vi "Diagnostic.vi"(8 "error in (no error)":errorcluster, 11 "Connection Data In":T1) -> (0 "error out":errorcluster, 3 "Connection Data Out":T1)   [LabVIEW 2014, in "MSX-E3711_dll.lvlib"]
doc: "Encargado de Testear si hay transductores desconectados, si se produjo un corto circuito en alguno de ellos y de rearmarlos."
uses:
  MSX-E3711_dll.lvlib
  Typedef/Connection Data.ctl
  E:/Repositorio Magnis/INF002/v0/Modules/HAL/Drivers/Sync/ADDI-DATA MSX-E3711/API/MSXE371x.dll
  MSXE371x.dll
  E:/Repositorio Magnis/INF002/v0/Modules/HAL/Drivers/Sync/ADDI-DATA MSX-E3711/API/MXCommon.dll
  MXCommon.dll
panel:
  out "String":string
  out "Rearm \nTransducers Status":bool
  out "Progress Status":i32(slide) scale=0.0..100.0
  out "Table":string[][](table)=[["-", "-"], ["-", "-"], ["-", "-"], ["-", "-"], ["-", "-"], ["-", "-"], ["-", "-"], ["-", "-"], ["-", "-"], ["-", "-"], ["-", "-"], ["-", "-"], ["-", "-"], ["-", "-"], ["-", "-"], ["-", "-"], ["-", "-"]]
  in  "Rearm Transducers":bool
  in  "ConnectionStatus":bool
  in  "ShortCircuit":bool
  in  "Start":bool
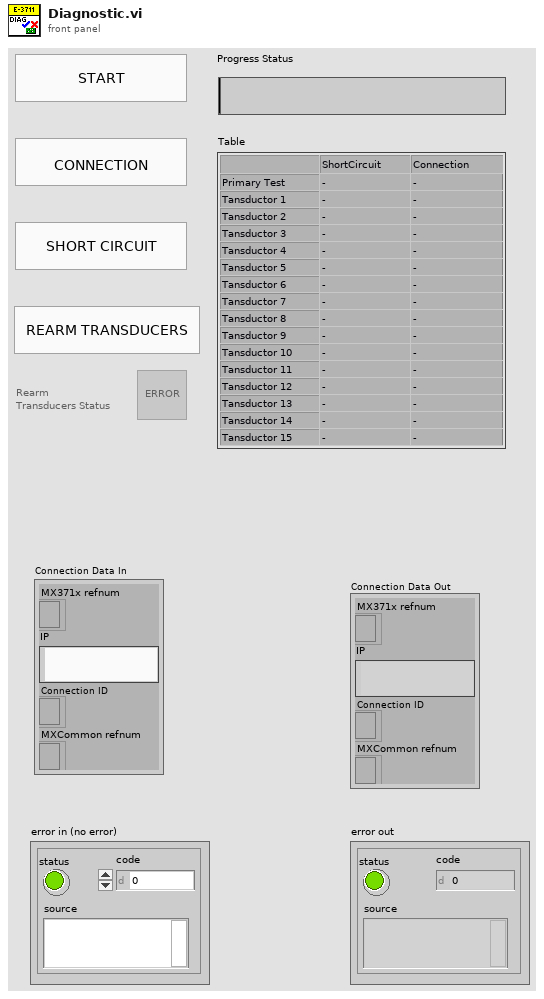
[diagram p1: front panel]
types:
  T1 = typedef "MSX-E3711_dll.lvlib/Connection Data.ctl" = cluster{"MX371x refnum":refnum<k24>, "IP":string, "Connection ID ":refnum<k5>, "MXCommon refnum":refnum<k24>}
  T2 = enum8{"Enabled", "Disabled", "Disabled and Grayed Out"}
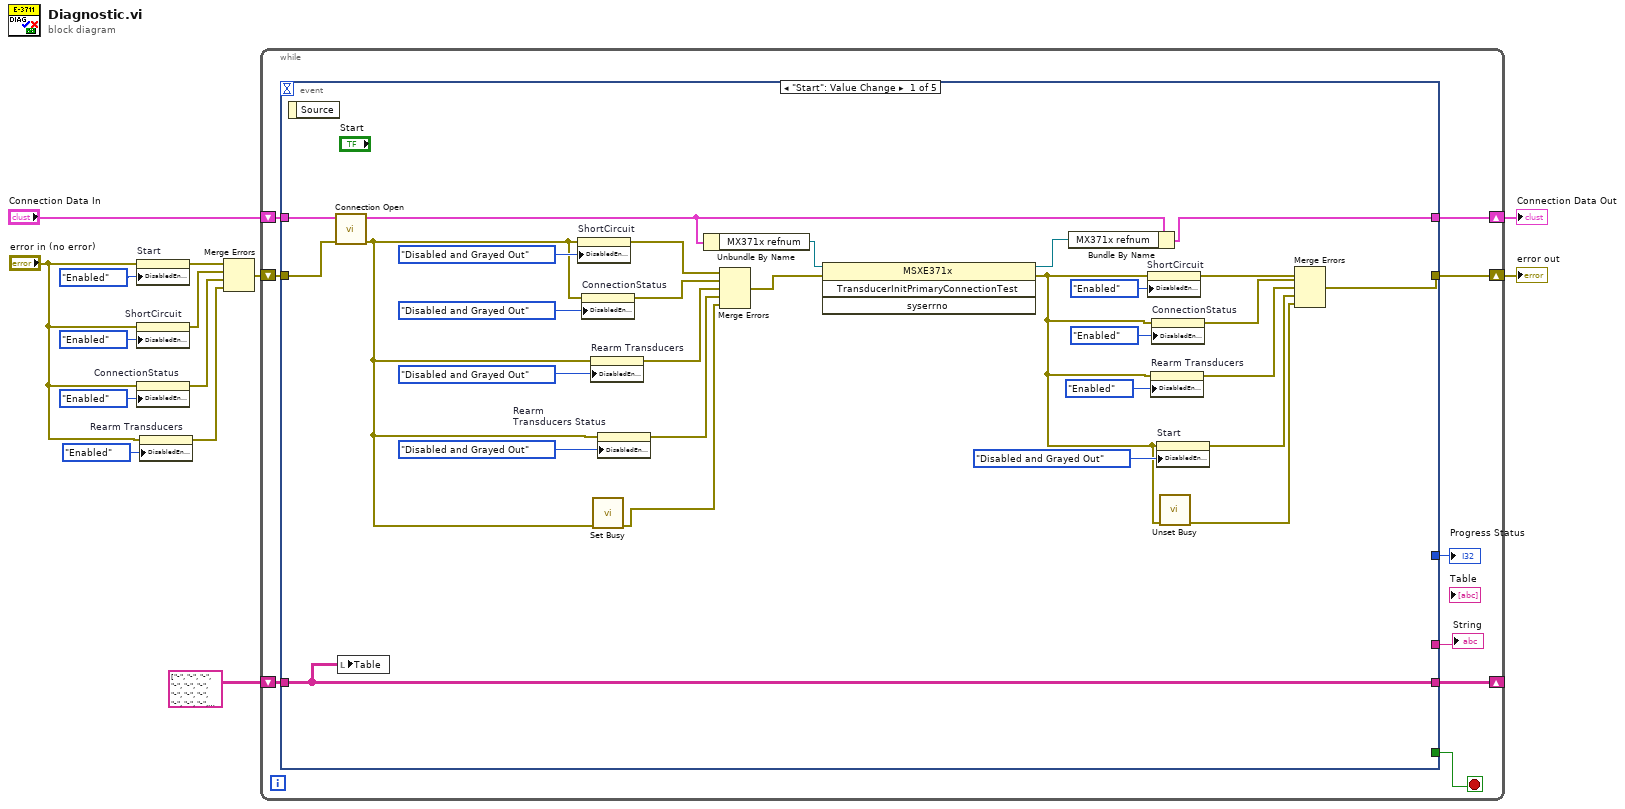
[diagram p0: block diagram]
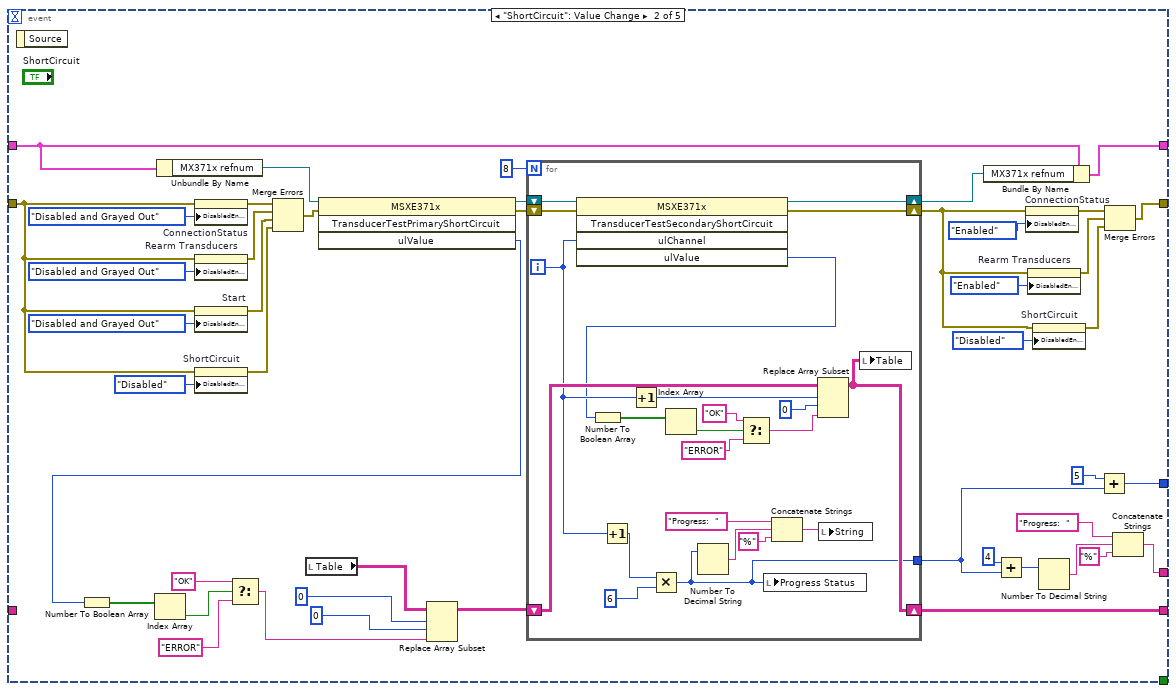
[diagram p2: hidden frame]
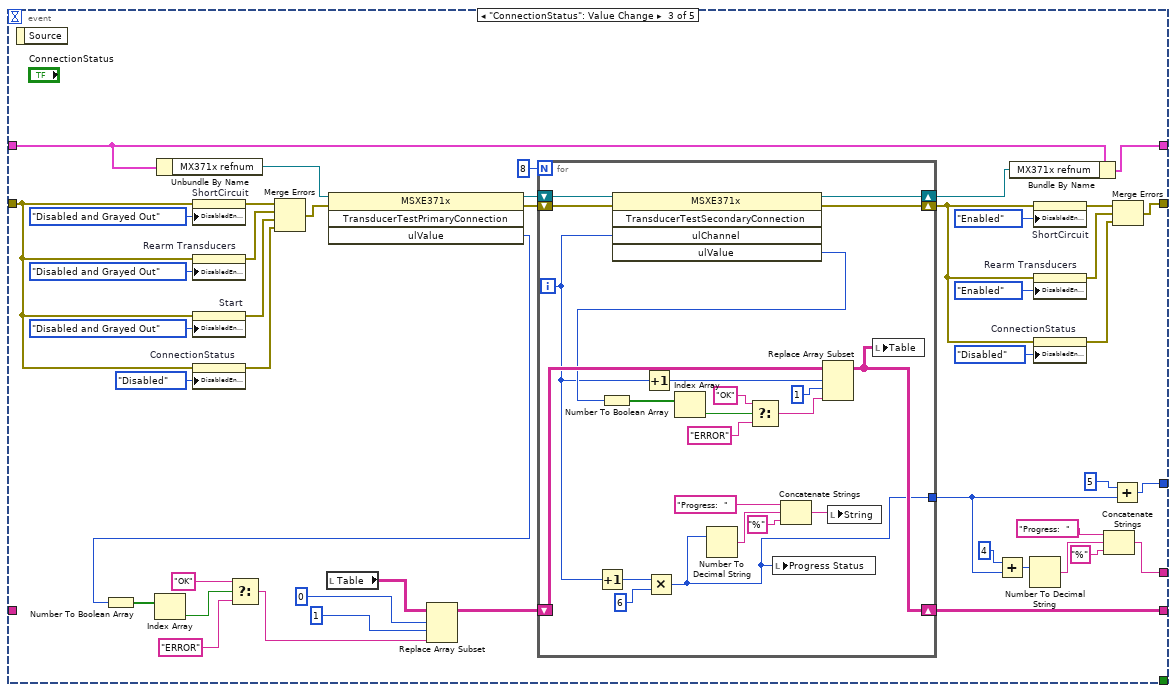
[diagram p3: hidden frame]
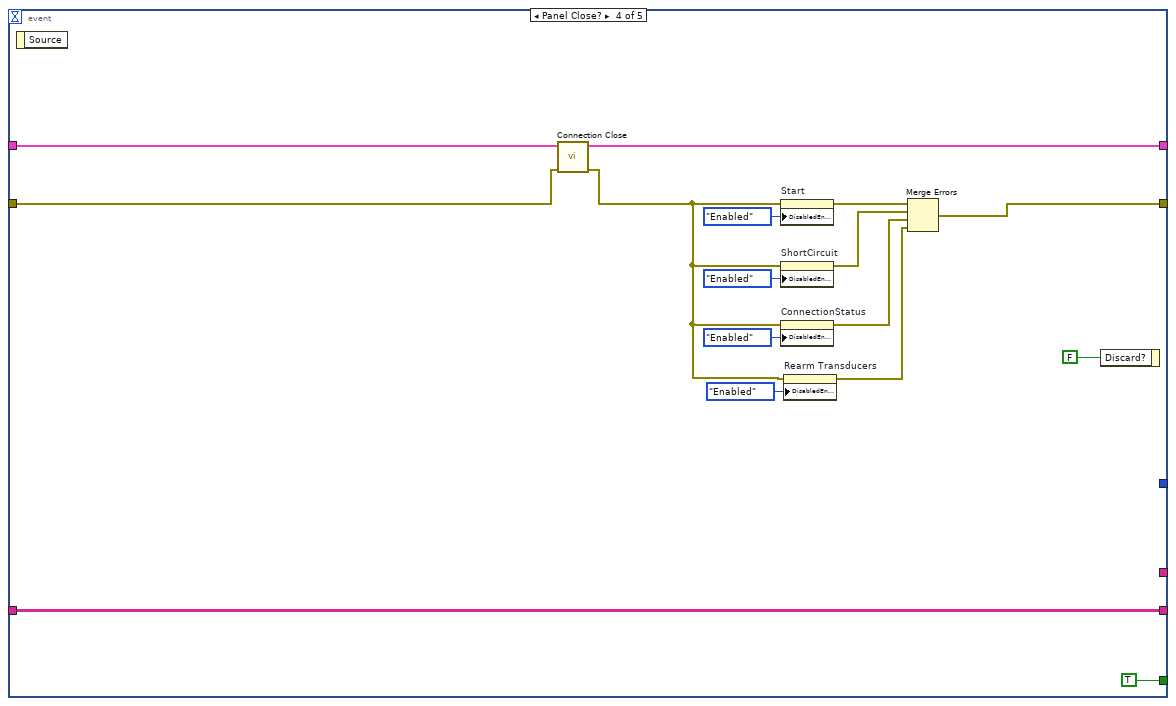
[diagram p4: hidden frame]
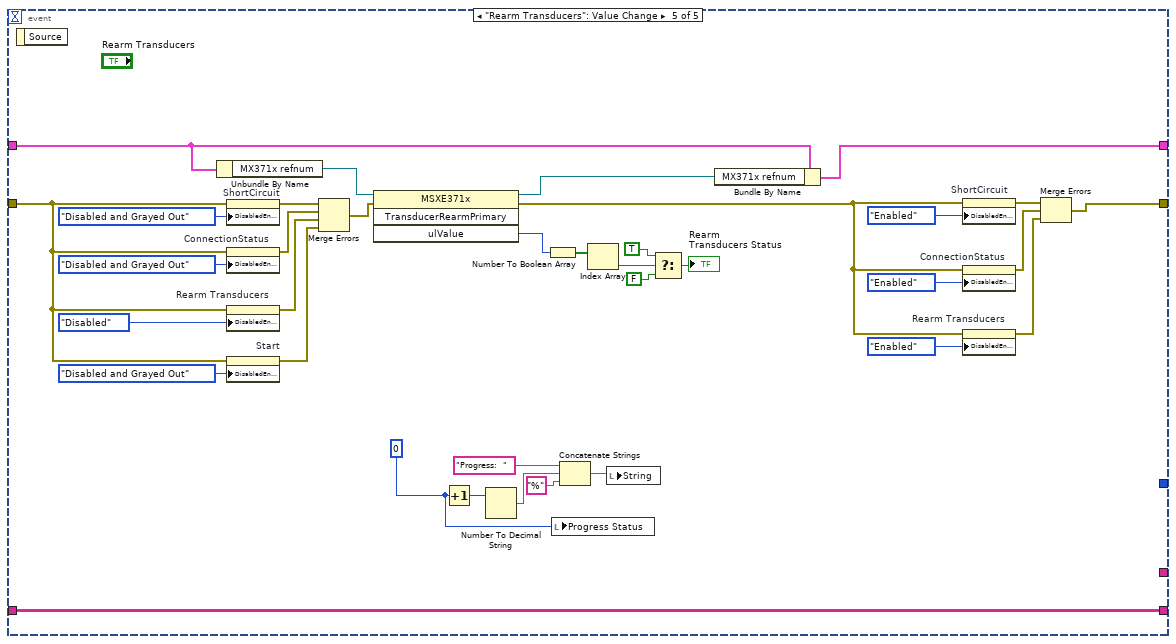
[diagram p5: hidden frame]
diagram:
  n1 = property on="Start" class="Bool"(error in="error in (no error)", "DisabledEnum"=T2."Enabled" ("Disabled")) -> (error out=w6:errorcluster)  [unwired: 1 in, 1 out]
  n2 = property on="ShortCircuit" class="Bool"(error in="error in (no error)", "DisabledEnum"=T2."Enabled" ("Disabled")) -> (error out=w7:errorcluster)  [unwired: 1 in, 1 out]
  n3 = property on="ConnectionStatus" class="Bool"(error in="error in (no error)", "DisabledEnum"=T2."Enabled" ("Disabled")) -> (error out=w8:errorcluster)  [unwired: 1 in, 1 out]
  n4 = property on="Rearm Transducers" class="Bool"(error in="error in (no error)", "DisabledEnum"=T2."Enabled" ("Disabled")) -> (error out=w10:errorcluster)  [unwired: 1 in, 1 out]
  n5 = Merge Errors(w6, w7, w8, w10) -> (w1:errorcluster)
  n6 = while {
    shift-right: [w22] -> w13
    shift-left: "Connection Data In" -> [w21]
    shift-right: [w19] -> w12
    shift-left: w1 -> [w20]
    shift-right: [w17] -> _
    shift-left: string[][] [["-", "-"], ["-", "-"], ["-", "-"], ["-", "-"], ["-", "-"], ["-", "-"], ["-", "-"], ["-", "-"], ["-", "-"]] ("Table") -> [w18]
    stop <- w23 stop-if-true
    n7 = event shown="[0] \"Start\": Value Change" {
      selector: _ -> [_ _ _ _ _]
      dyn-events: _ -> [_ _ _ _ _]
      timeout: _ -> [_ _ _ _ _]
      tunnel: [_ _ _ TRUE ("Close") _] -> w23
      tunnel: [w52 w75 w162 w198 w236] -> w22
      tunnel: w21 -> [w51 w85 w163 w199 w237]
      tunnel: [w41 w76 w141 w190 w226] -> w19
      tunnel: w20 -> [w49 w61 w129 w197 w210]
      tunnel: w18 -> [w40 _ _ w202 w235]
      tunnel: [_ w67 w158 _ _] -> w15
      tunnel: [w40 w86 w147 w202 w235] -> w17
      tunnel: [_ w68 w136 _ _] -> w16
      event "Start": Value Change {
        n8 = event-data() -> ()  [unwired: 1 in, 1 out]
        n9 = call "Connection Open.vi"("error in (no error)"=w49, "Connection Data In"=w51) -> ("error out"=w30:errorcluster, "Connection Data Out"=w50:T1)  [unwired: 8 in]
        n10 = local write "Table"(w40) -> ()
        n11 = property on="ShortCircuit" class="Bool"(error in=w30, "DisabledEnum"=T2."Disabled and Grayed Out" ("Disabled")) -> (error out=w48:errorcluster)  [unwired: 1 in, 1 out]
        n12 = property on="ConnectionStatus" class="Bool"(error in=w30, "DisabledEnum"=T2."Disabled and Grayed Out" ("Disabled")) -> (error out=w38:errorcluster)  [unwired: 1 in, 1 out]
        n13 = property on="Rearm Transducers" class="Bool"(error in=w30, "DisabledEnum"=T2."Disabled and Grayed Out" ("Disabled")) -> (error out=w37:errorcluster)  [unwired: 1 in, 1 out]
        n14 = call <vilib>:"Set Busy.vi"("error in (no error)"=w30) -> ("error out"=w29:errorcluster)  [unwired: 9 in, 1 out]
        n15 = property on="Rearm \nTransducers Status" class="Bool (strict)"(error in=w30, "DisabledEnum"=T2."Disabled and Grayed Out" ("Disabled")) -> (error out=w31:errorcluster)  [unwired: 1 in, 1 out]
        n16 = Unbundle By Name(w50) -> ("MX371x refnum"=w24:refnum<k24>)
        n17 = Merge Errors(w48, w38, w37, w31, w29) -> (w25:errorcluster)
        n18 = invoke class="MSXE371x" method="TransducerInitPrimaryConnectionTest"(reference=w24, error in=w25) -> (reference out=w27:refnum<k24>, error out=w26:errorcluster)  [unwired: 2 in, 2 out]
        n19 = Bundle By Name(cluster=w50, "MX371x refnum"=w27) -> (w52:T1)
        n20 = property on="ShortCircuit" class="Bool"(error in=w26, "DisabledEnum"=T2."Enabled" ("Disabled")) -> (error out=w42:errorcluster)  [unwired: 1 in, 1 out]
        n21 = property on="Rearm Transducers" class="Bool"(error in=w26, "DisabledEnum"=T2."Enabled" ("Disabled")) -> (error out=w35:errorcluster)  [unwired: 1 in, 1 out]
        n22 = property on="ConnectionStatus" class="Bool"(error in=w26, "DisabledEnum"=T2."Enabled" ("Disabled")) -> (error out=w45:errorcluster)  [unwired: 1 in, 1 out]
        n23 = property on="Start" class="Bool"(error in=w26, "DisabledEnum"=T2."Disabled and Grayed Out" ("Disabled")) -> (error out=w33:errorcluster)  [unwired: 1 in, 1 out]
        n24 = call <vilib>:"Unset Busy.vi"("error in (no error)"=w26) -> ("error out"=w28:errorcluster)  [unwired: 10 in]
        n25 = Merge Errors(w42, w45, w35, w33, w28) -> (w41:errorcluster)
      }
      event "ShortCircuit": Value Change {
        n26 = event-data() -> ()  [unwired: 1 in, 1 out]
        n27 = Unbundle By Name(w85) -> ("MX371x refnum"=w54:refnum<k24>)
        n28 = property on="ConnectionStatus" class="Bool"(error in=w61, "DisabledEnum"=T2."Disabled and Grayed Out" ("Disabled")) -> (error out=w82:errorcluster)  [unwired: 1 in, 1 out]
        n29 = property on="Rearm Transducers" class="Bool"(error in=w61, "DisabledEnum"=T2."Disabled and Grayed Out" ("Disabled")) -> (error out=w81:errorcluster)  [unwired: 1 in, 1 out]
        n30 = property on="Start" class="Bool"(error in=w61, "DisabledEnum"=T2."Disabled and Grayed Out" ("Disabled")) -> (error out=w63:errorcluster)  [unwired: 1 in, 1 out]
        n31 = property on="ShortCircuit" class="Bool"(error in=w61, "DisabledEnum"=T2."Disabled" ("Disabled")) -> (error out=w62:errorcluster)  [unwired: 1 in, 1 out]
        n32 = Merge Errors(w82, w81, w63, w62) -> (w57:errorcluster)
        n33 = local read "Table"() -> (w91:string[][])
        n34 = invoke class="MSXE371x" method="TransducerTestPrimaryShortCircuit"(reference=w54, error in=w57) -> (reference out=w55:refnum<k24>, error out=w56:errorcluster, "ulValue"=w53:u64)  [unwired: 2 in, 1 out]
        n35 = Number To Boolean Array(number=w53) -> (Boolean array=w97:bool[])
        n36 = Index Array(array=w97) -> (element=w96:bool)  [unwired: 1 in]
        n37 = Select(t="OK" ("String"), s=w96, f="ERROR" ("String")) -> (s? t:f=w88:string)
        n38 = Replace Array Subset(array=w91, new element=w88, index (row)=0, index (col)=0 ("disabled index (col)")) -> (w87:string[][])
        n39 = for {
          N: 8 -> [_]
          shift-right: [w99] -> w92
          shift-left: w55 -> [w103]
          shift-right: [w98] -> w59
          shift-left: w56 -> [w102]
          shift-right: [w107] -> w86
          shift-left: w87 -> [w108]
          tunnel: [w104] -> w66
          i -> [w101]
          n40 = invoke class="MSXE371x" method="TransducerTestSecondaryShortCircuit"(reference=w103, error in=w102, "ulChannel"=w101) -> (reference out=w99:refnum<k24>, error out=w98:errorcluster, "ulValue"=w100:u64)  [unwired: 2 in, 2 out]
          n41 = Number To Boolean Array(number=w100) -> (Boolean array=w119:bool[])
          n42 = Increment(x=w101) -> (x+1=w106:i32)
          n43 = Increment(x=w101) -> (x+1=w111:i32)
          n44 = Multiply(x=w106, y=6) -> (x*y=w104:i32)
          n45 = Index Array(array=w119) -> (element=w118:bool)  [unwired: 1 in]
          n46 = Number To Decimal String(number=w104) -> (decimal integer string=w113:string)  [unwired: 1 out]
          n47 = Select(t="OK" ("String"), s=w118, f="ERROR" ("String")) -> (s? t:f=w109:string)
          n48 = local write "Progress Status"(w104) -> ()
          n49 = Concatenate Strings("Progress:  ", w113, "%") -> (w115:string)
          n50 = Replace Array Subset(array=w108, new element=w109, index (row)=w111, index (col)=0) -> (w107:string[][])
          n51 = local write "String"(w115) -> ()
          n52 = local write "Table"(w107) -> ()
        }
        n53 = Bundle By Name(cluster=w85, "MX371x refnum"=w92) -> (w75:T1)
        n54 = Add(x=4, y=w66) -> (x+y=w69:i32)
        n55 = property on="ConnectionStatus" class="Bool"(error in=w59, "DisabledEnum"=T2."Enabled" ("Disabled")) -> (error out=w77:errorcluster)  [unwired: 1 in, 1 out]
        n56 = property on="Rearm Transducers" class="Bool"(error in=w59, "DisabledEnum"=T2."Enabled" ("Disabled")) -> (error out=w78:errorcluster)  [unwired: 1 in, 1 out]
        n57 = property on="ShortCircuit" class="Bool"(error in=w59, "DisabledEnum"=T2."Disabled" ("Disabled")) -> (error out=w58:errorcluster)  [unwired: 1 in, 1 out]
        n58 = Number To Decimal String(number=w69) -> (decimal integer string=w72:string)  [unwired: 1 out]
        n59 = Add(x=5, y=w66) -> (x+y=w67:i32)
        n60 = Merge Errors(w77, w78, w58) -> (w76:errorcluster)
        n61 = Concatenate Strings("Progress:  ", w72, "%") -> (w68:string)
      }
      event "ConnectionStatus": Value Change {
        n62 = event-data() -> ()  [unwired: 1 in, 1 out]
        n63 = Unbundle By Name(w163) -> ("MX371x refnum"=w121:refnum<k24>)
        n64 = property on="ShortCircuit" class="Bool"(error in=w129, "DisabledEnum"=T2."Disabled and Grayed Out" ("Disabled")) -> (error out=w145:errorcluster)  [unwired: 1 in, 1 out]
        n65 = property on="Rearm Transducers" class="Bool"(error in=w129, "DisabledEnum"=T2."Disabled and Grayed Out" ("Disabled")) -> (error out=w144:errorcluster)  [unwired: 1 in, 1 out]
        n66 = property on="Start" class="Bool"(error in=w129, "DisabledEnum"=T2."Disabled and Grayed Out" ("Disabled")) -> (error out=w130:errorcluster)  [unwired: 1 in, 1 out]
        n67 = property on="ConnectionStatus" class="Bool"(error in=w129, "DisabledEnum"=T2."Disabled" ("Disabled")) -> (error out=w128:errorcluster)  [unwired: 1 in, 1 out]
        n68 = Merge Errors(w145, w144, w130, w128) -> (w122:errorcluster)
        n69 = local read "Table"() -> (w153:string[][])
        n70 = invoke class="MSXE371x" method="TransducerTestPrimaryConnection"(reference=w121, error in=w122) -> (reference out=w124:refnum<k24>, error out=w123:errorcluster, "ulValue"=w120:u64)  [unwired: 2 in, 1 out]
        n71 = Number To Boolean Array(number=w120) -> (Boolean array=w149:bool[])
        n72 = Index Array(array=w149) -> (element=w150:bool)  [unwired: 1 in]
        n73 = Select(t="OK" ("String"), s=w150, f="ERROR" ("String")) -> (s? t:f=w156:string)
        n74 = Replace Array Subset(array=w153, new element=w156, index (row)=0, index (col)=1 ("disabled index (col)")) -> (w148:string[][])
        n75 = for {
          N: 8 -> [_]
          shift-right: [w169] -> w125
          shift-left: w123 -> [w165]
          shift-right: [w170] -> w164
          shift-left: w124 -> [w166]
          shift-right: [w174] -> w147
          shift-left: w148 -> [w175]
          tunnel: [w171] -> w134
          i -> [w167]
          n76 = Increment(x=w167) -> (x+1=w173:i32)
          n77 = invoke class="MSXE371x" method="TransducerTestSecondaryConnection"(reference=w166, error in=w165, "ulChannel"=w167) -> (reference out=w170:refnum<k24>, error out=w169:errorcluster, "ulValue"=w168:u64)  [unwired: 2 in, 2 out]
          n78 = Number To Boolean Array(number=w168) -> (Boolean array=w176:bool[])
          n79 = Increment(x=w167) -> (x+1=w184:i32)
          n80 = Multiply(x=w173, y=6) -> (x*y=w171:i32)
          n81 = Index Array(array=w176) -> (element=w177:bool)  [unwired: 1 in]
          n82 = Number To Decimal String(number=w171) -> (decimal integer string=w182:string)  [unwired: 1 out]
          n83 = Select(t="OK" ("String"), s=w177, f="ERROR" ("String")) -> (s? t:f=w186:string)
          n84 = local write "Progress Status"(w171) -> ()
          n85 = Concatenate Strings("Progress:  ", w182, "%") -> (w180:string)
          n86 = Replace Array Subset(array=w175, new element=w186, index (row)=w184, index (col)=1) -> (w174:string[][])
          n87 = local write "String"(w180) -> ()
          n88 = local write "Table"(w174) -> ()
        }
        n89 = Add(x=4, y=w134) -> (x+y=w133:i32)
        n90 = Bundle By Name(cluster=w163, "MX371x refnum"=w164) -> (w162:T1)
        n91 = Number To Decimal String(number=w133) -> (decimal integer string=w138:string)  [unwired: 1 out]
        n92 = property on="ShortCircuit" class="Bool"(error in=w125, "DisabledEnum"=T2."Enabled" ("Disabled")) -> (error out=w140:errorcluster)  [unwired: 1 in, 1 out]
        n93 = property on="Rearm Transducers" class="Bool"(error in=w125, "DisabledEnum"=T2."Enabled" ("Disabled")) -> (error out=w142:errorcluster)  [unwired: 1 in, 1 out]
        n94 = property on="ConnectionStatus" class="Bool"(error in=w125, "DisabledEnum"=T2."Disabled" ("Disabled")) -> (error out=w126:errorcluster)  [unwired: 1 in, 1 out]
        n95 = Concatenate Strings("Progress:  ", w138, "%") -> (w136:string)
        n96 = Add(x=5, y=w134) -> (x+y=w158:i32)
        n97 = Merge Errors(w140, w142, w126) -> (w141:errorcluster)
      }
      event Panel Close? {
        n98 = event-data() -> ()  [unwired: 1 in, 1 out]
        n99 = call "Connection Close.vi"("error in (no error)"=w197, "Connection Data In"=w199) -> ("error out"=w187:errorcluster, "Connection Data Out"=w198:T1)  [unwired: 8 in]
        n100 = property on="Start" class="Bool"(error in=w187, "DisabledEnum"=T2."Enabled" ("Disabled")) -> (error out=w193:errorcluster)  [unwired: 1 in, 1 out]
        n101 = property on="ShortCircuit" class="Bool"(error in=w187, "DisabledEnum"=T2."Enabled" ("Disabled")) -> (error out=w192:errorcluster)  [unwired: 1 in, 1 out]
        n102 = property on="ConnectionStatus" class="Bool"(error in=w187, "DisabledEnum"=T2."Enabled" ("Disabled")) -> (error out=w191:errorcluster)  [unwired: 1 in, 1 out]
        n103 = property on="Rearm Transducers" class="Bool"(error in=w187, "DisabledEnum"=T2."Enabled" ("Disabled")) -> (error out=w188:errorcluster)  [unwired: 1 in, 1 out]
        n104 = Merge Errors(w193, w192, w191, w188) -> (w190:errorcluster)
        n105 = event-data("Discard?"=FALSE) -> ()  [unwired: 1 in, 1 out]
      }
      event "Rearm Transducers": Value Change {
        w218 = 0
        n106 = event-data() -> ()  [unwired: 1 in, 1 out]
        n107 = Unbundle By Name(w237) -> ("MX371x refnum"=w203:refnum<k24>)
        n108 = property on="ShortCircuit" class="Bool"(error in=w210, "DisabledEnum"=T2."Disabled and Grayed Out" ("Disabled")) -> (error out=w223:errorcluster)  [unwired: 1 in, 1 out]
        n109 = property on="ConnectionStatus" class="Bool"(error in=w210, "DisabledEnum"=T2."Disabled and Grayed Out" ("Disabled")) -> (error out=w222:errorcluster)  [unwired: 1 in, 1 out]
        n110 = property on="Rearm Transducers" class="Bool"(error in=w210, "DisabledEnum"=T2."Disabled" ("Disabled")) -> (error out=w213:errorcluster)  [unwired: 1 in, 1 out]
        n111 = property on="Start" class="Bool"(error in=w210, "DisabledEnum"=T2."Disabled and Grayed Out" ("Disabled")) -> (error out=w211:errorcluster)  [unwired: 1 in, 1 out]
        n112 = Merge Errors(w223, w222, w213, w211) -> (w207:errorcluster)
        n113 = invoke class="MSXE371x" method="TransducerRearmPrimary"(reference=w203, error in=w207) -> (reference out=w205:refnum<k24>, error out=w206:errorcluster, "ulValue"=w204:u64)  [unwired: 2 in, 1 out]
        n114 = Increment(x=w218) -> (x+1=w219:i32)
        n115 = Number To Decimal String(number=w219) -> (decimal integer string=w231:string)  [unwired: 1 out]
        n116 = Number To Boolean Array(number=w204) -> (Boolean array=w234:bool[])
        n117 = local write "Progress Status"(w218) -> ()
        n118 = Concatenate Strings("Progress:  ", w231, "%") -> (w229:string)
        n119 = Index Array(array=w234) -> (element=w233:bool)  [unwired: 1 in]
        n120 = local write "String"(w229) -> ()
        n121 = Select(t=TRUE, s=w233, f=FALSE) -> (s? t:f=→"Rearm \nTransducers Status":bool)
        n122 = Bundle By Name(cluster=w237, "MX371x refnum"=w205) -> (w236:T1)
        n123 = property on="ShortCircuit" class="Bool"(error in=w206, "DisabledEnum"=T2."Enabled" ("Disabled")) -> (error out=w228:errorcluster)  [unwired: 1 in, 1 out]
        n124 = property on="ConnectionStatus" class="Bool"(error in=w206, "DisabledEnum"=T2."Enabled" ("Disabled")) -> (error out=w227:errorcluster)  [unwired: 1 in, 1 out]
        n125 = property on="Rearm Transducers" class="Bool"(error in=w206, "DisabledEnum"=T2."Enabled" ("Disabled")) -> (error out=w208:errorcluster)  [unwired: 1 in, 1 out]
        n126 = Merge Errors(w228, w227, w208) -> (w226:errorcluster)
      }
    }
    "String" <- w16
    "Progress Status" <- w15
  }
  "error out" <- w12
  "Connection Data Out" <- w13
